vi "m10.wf.compose.vi"(0 "Waveform In":waveform(dbl), 2 "Repetitions":T1 {"Rep type" items=["Off", "DC", "Trig", "Train", "Gate"]}, 11 "error in (no error)":errorcluster) -> (4 "Analog Waveform Out":waveform(dbl), 6 "Digital Waveform Out":digitalwaveform(waveform), 15 "error out":errorcluster)   [LabVIEW 2009]
uses:
  <vilib>/Waveform/WDTOps.llb/WDT Waveform Duration DBL.vi
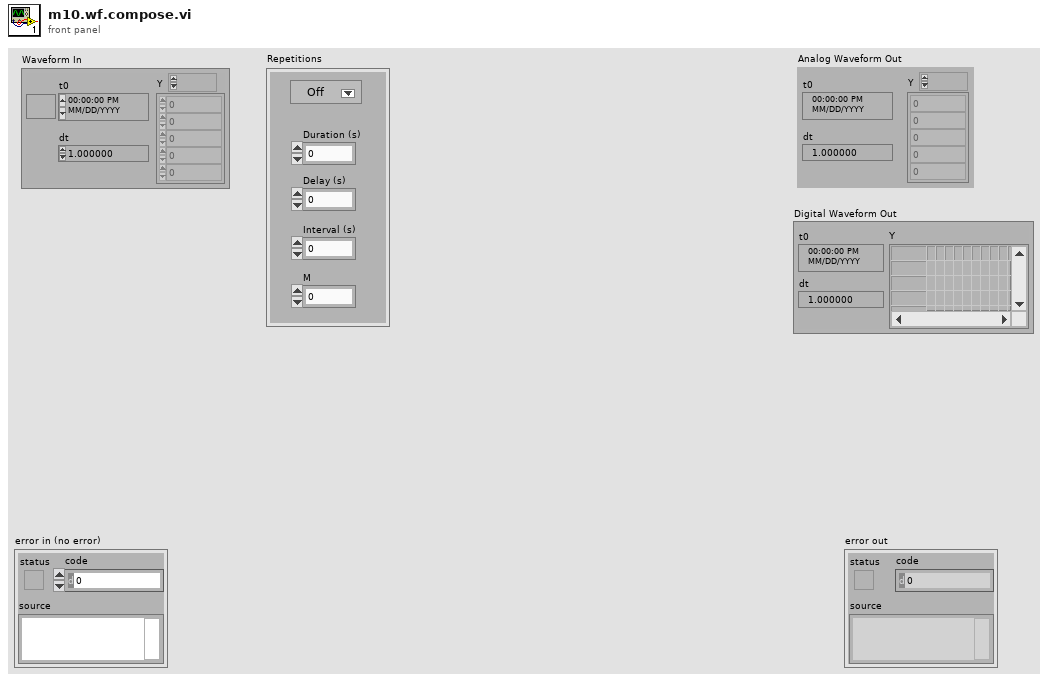
[diagram p1: front panel]
types:
  T1 = cluster{"Rep type":u16, "Duration (s)":dbl, "Delay (s)":dbl, "Interval (s)":dbl, "M":i32}
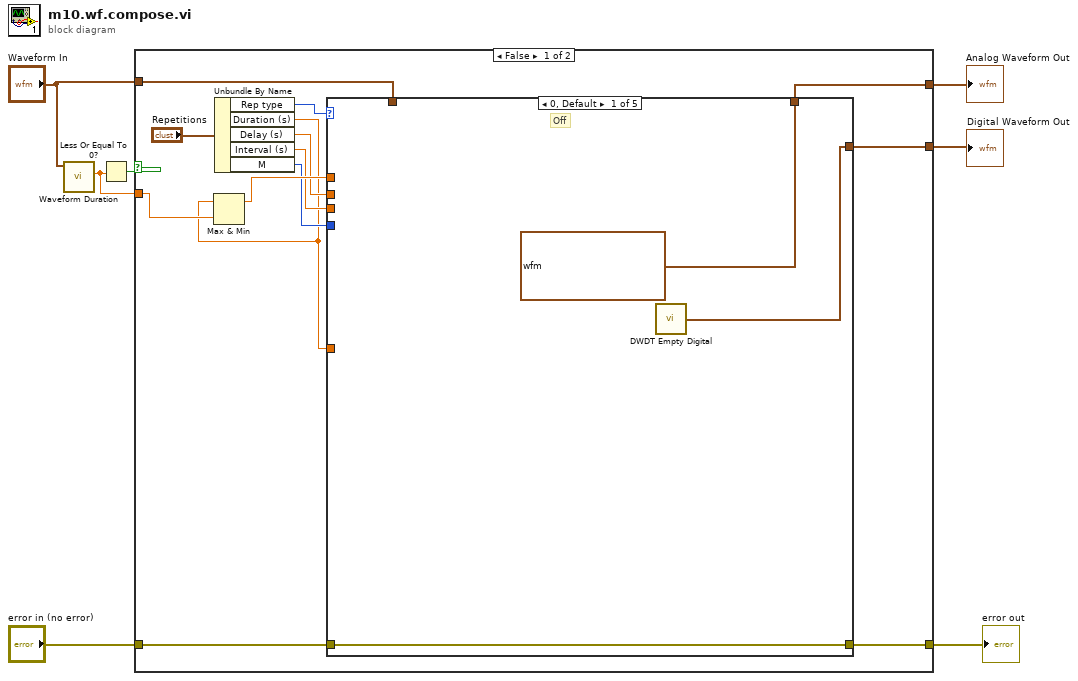
[diagram p0: block diagram]
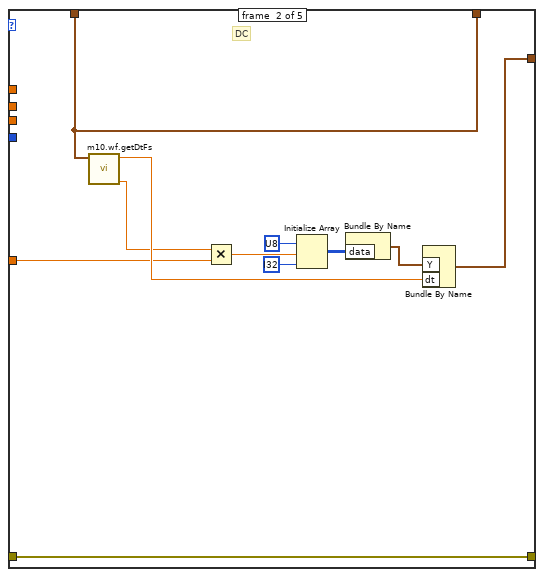
[diagram p2: hidden frame]
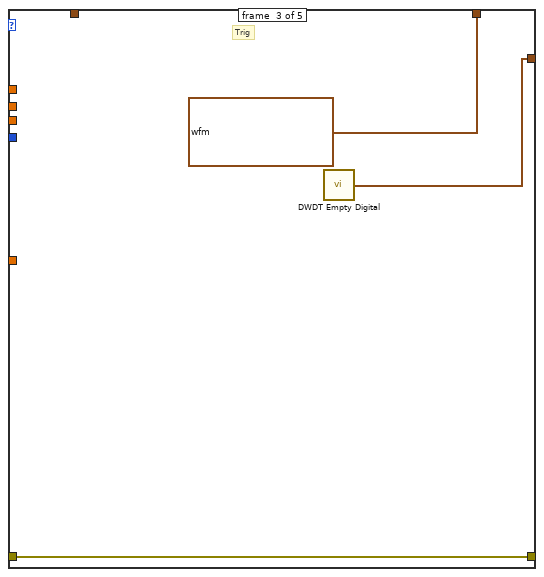
[diagram p3: hidden frame]
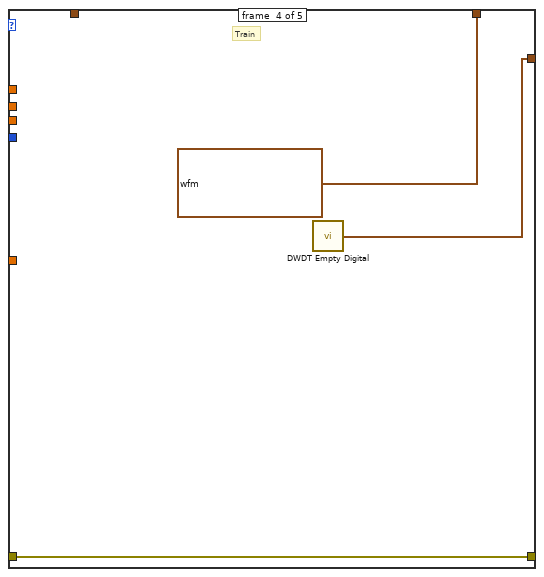
[diagram p4: hidden frame]
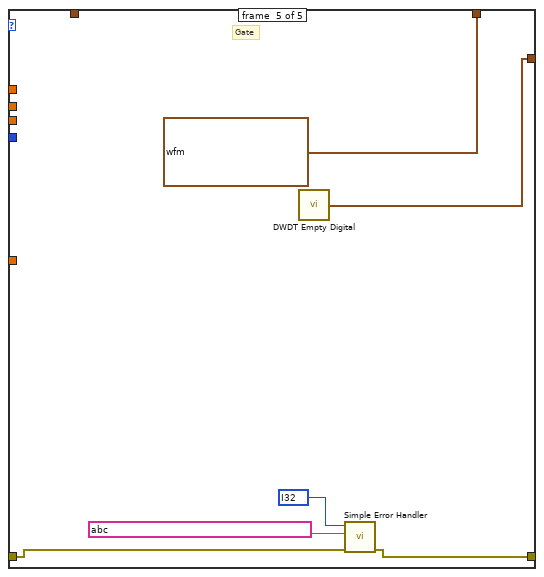
[diagram p5: hidden frame]
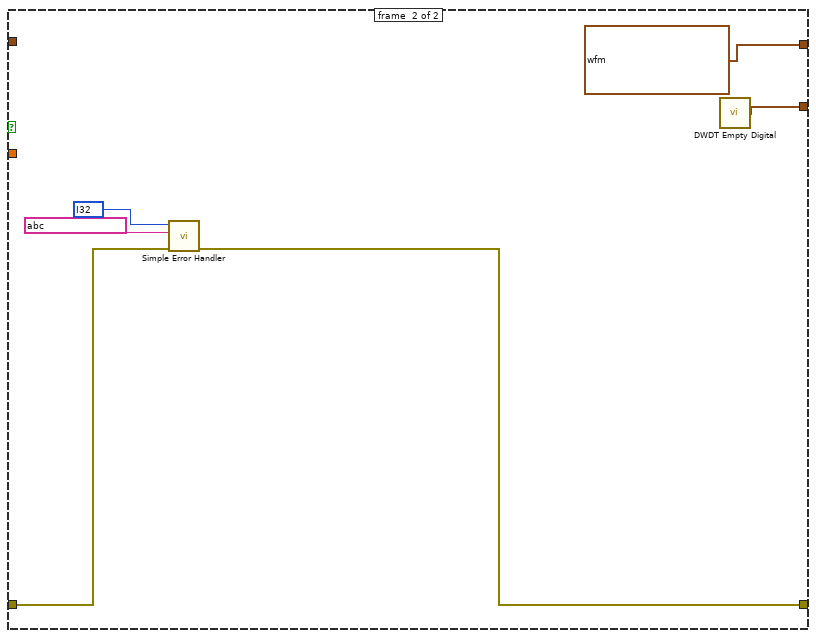
[diagram p6: hidden frame]
diagram:
  n1 = call-poly <vilib>:"Waveform Duration.vi"("waveform in"="Waveform In") -> ("duration"=w4:dbl)  [unwired: 8 in, 2 out]
  n2 = Less Or Equal To 0?(x=w4) -> (x <= 0?=w7:bool)
  n3 = case shown="False" w7 {
    tunnel: "error in (no error)" -> [w13 w52]
    tunnel: [w12 w49] -> w5
    tunnel: w4 -> [w19 _]
    tunnel: "Waveform In" -> [w11 _]
    tunnel: [w10 waveform(dbl) ? ("Waveform")] -> w2
    tunnel: [w8 w48] -> w1
    frame #0 {
      n4 = Unbundle By Name("Repetitions") -> ("Rep type"=w18:u16, "Duration (s)"=w9:dbl, "Delay (s)"=w16:dbl, "Interval (s)"=w15:dbl, "M"=w14:i32)
      n5 = Max & Min(x=w9, y=w19) -> (max(x,y)=w17:dbl)  [unwired: 1 out]
      n6 = case shown="0, Default" w18 {
        tunnel: w17 -> [_ _ _ _ _]
        tunnel: w16 -> [_ _ _ _ _]
        tunnel: w15 -> [_ _ _ _ _]
        tunnel: w14 -> [_ _ _ _ _]
        tunnel: w13 -> [w21 w28 w35 w40 w46]
        tunnel: [w21 w28 w35 w40 w44] -> w12
        tunnel: w11 -> [_ w34 _ _ _]
        tunnel: [waveform(dbl) ? ("Waveform") w34 waveform(dbl) ? ("Waveform") waveform(dbl) ? ("Waveform") waveform(dbl) ? ("Waveform")] -> w10
        tunnel: w9 -> [_ w25 _ _ _]
        tunnel: [w22 w29 w36 w38 w41] -> w8
        frame #0 {
          # "Off"
          n7 = call <vilib>:"DWDT Empty Digital.vi"() -> ("digital waveform out"=w22:digitalwaveform)  [unwired: 5 in]
        }
        frame #1 {
          # "DC"
          n8 = call "m10.wf.getDtFs.vi"("Waveform"=w34) -> ("Fs (Hz)"=w24:dbl, "dt"=w27:dbl)  [unwired: 9 in]
          n9 = Multiply(x=w24, y=w25) -> (x*y=w26:dbl)
          n10 = Initialize Array(u8 ? ("element"), w26, i32 ? ("dimension size")) -> (w31:u8[][])
          n11 = Bundle By Name("data"=w31) -> (w33:digitaldata)  [unwired: 1 in]
          n12 = Bundle By Name("Y"=w33, "dt"=w27) -> (w29:digitalwaveform)  [unwired: 1 in]
        }
        frame #2 {
          # "Trig"
          n13 = call <vilib>:"DWDT Empty Digital.vi"() -> ("digital waveform out"=w36:digitalwaveform)  [unwired: 5 in]
        }
        frame #3 {
          # "Train"
          n14 = call <vilib>:"DWDT Empty Digital.vi"() -> ("digital waveform out"=w38:digitalwaveform)  [unwired: 5 in]
        }
        frame #4 {
          # "Gate"
          n15 = call <vilib>:"DWDT Empty Digital.vi"() -> ("digital waveform out"=w41:digitalwaveform)  [unwired: 5 in]
          n16 = call <vilib>:"Simple Error Handler.vi"("error code (no error:0)"=i32 ?, "error source (\" \")"=string ? ("error source (\" \")"), "error in (no error)"=w46) -> ("error out"=w44:errorcluster)  [unwired: 2 in, 4 out]
        }
      }
    }
    frame #1 {
      n17 = call <vilib>:"Simple Error Handler.vi"("error code (no error:0)"=i32 ?, "error source (\" \")"=string ? ("error source (\" \")"), "error in (no error)"=w52) -> ("error out"=w49:errorcluster)  [unwired: 2 in, 4 out]
      n18 = call <vilib>:"DWDT Empty Digital.vi"() -> ("digital waveform out"=w48:digitalwaveform)  [unwired: 5 in]
    }
  }
  "error out" <- w5
  "Analog Waveform Out" <- w2
  "Digital Waveform Out" <- w1
